vi "Read defensive_plays.vi"(8 "error in (no error)":errorcluster, 11 "Playbook in":refnum<class "Playbook.lvclass">) -> (0 "error out":errorcluster, 2 "defensive_plays":T1, 3 "Playbook out":refnum<class "Playbook.lvclass">)   [LabVIEW 2023, in "Playbook.lvclass"]
uses:
  Playbook.lvclass
  deffensive_plays.ctl
  Play_class/Play.lvclass
  TestPlay_class/TestPlay.lvclass
  NormalDefensivePlay_class/NormalDefensivePlay.lvclass
  NormalDefensiveWithDuelistPlay_class/NormalDefensiveWithDuelistPlay.lvclass
  Playbook.lvclass/Playbook.ctl
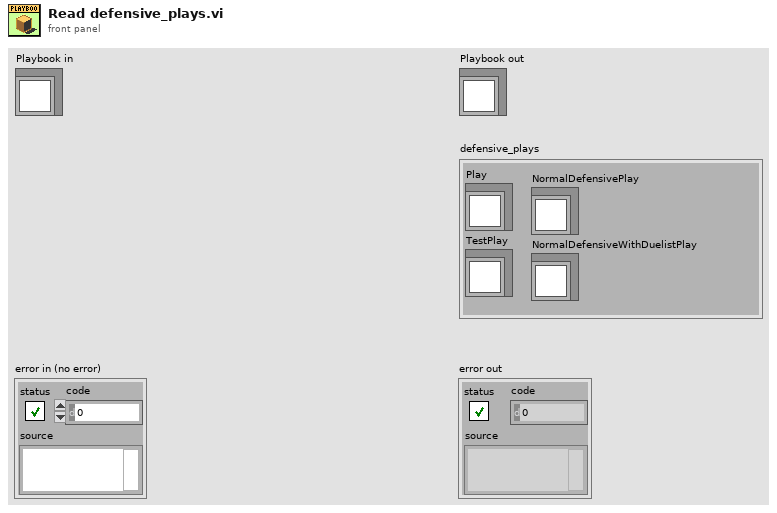
[diagram p1: front panel]
types:
  T1 = typedef "deffensive_plays.ctl" = cluster{"Play":refnum<class "Play.lvclass">, "TestPlay":refnum<class "TestPlay.lvclass">, "NormalDefensivePlay":refnum<class "NormalDefensivePlay.lvclass">, "NormalDefensiveWithDuelistPlay":refnum<class "NormalDefensiveWithDuelistPlay.lvclass">}
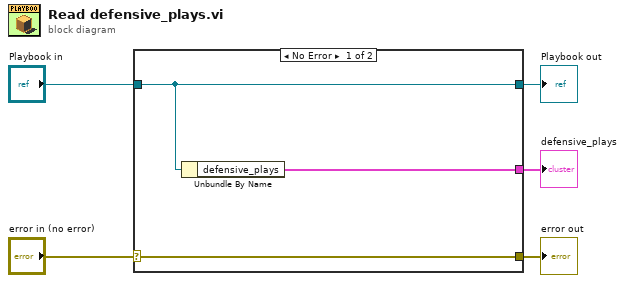
[diagram p0: block diagram]
diagram:
  n1 = case shown="No Error" "error in (no error)" {
    selector: "error in (no error)" -> [w8 w9]
    tunnel: [w8 w9] -> w4
    tunnel: [w7 w10] -> w2
    tunnel: "Playbook in" -> [w7 w10]
    tunnel: [w6 _] -> w1
    frame No Error {
      n2 = Unbundle By Name(w7) -> ("defensive_plays"=w6:T1)
    }
    frame Error {
    }
  }
  "error out" <- w4
  "Playbook out" <- w2
  "defensive_plays" <- w1
